vi "APU 1.4 In Place Output Read Structure.vi"(7 "Device outputs in":dbl[](array[numeric]), 8 "error in (no error)":errorcluster, 9 "FPGA ref in":T1, 11 "1.4 APU in":T4={"register names"={"shared settings"="", "input"="", "settings"="", "output"="", "go"="", "master"="", "send trigger"=""}, "shared settings"={"start"=0.0, "stuck limit"=0.0}, "settings"={"acceleration"=0.0, "enable accel"=FALSE}, "FIFO indexes"={"inputs"={"desired speed"=0, "reset"=0}, "outputs"={"crank angle"=0, "cycle angle"=0, "actual speed"=0, "devices synchronized"=0, "deviation error"=0}}, "input"={"desired speed"=0.0, "reset"=TRUE}, "degrees of 1 cycle u16"=0.0, "degrees of 1 crank u16"=0.0, "max deviation angle"=0.0}) -> (0 "error out":errorcluster, 1 "FPGA ref out":T1, 3 "1.4 APU out":T4={"register names"={"shared settings"="", "input"="", "settings"="", "output"="", "go"="", "master"="", "send trigger"=""}, "shared settings"={"start"=0.0, "stuck limit"=0.0}, "settings"={"acceleration"=0.0, "enable accel"=FALSE}, "FIFO indexes"={"inputs"={"desired speed"=0, "reset"=0}, "outputs"={"crank angle"=0, "cycle angle"=0, "actual speed"=0, "devices synchronized"=0, "deviation error"=0}}, "input"={"desired speed"=0.0, "reset"=TRUE}, "degrees of 1 cycle u16"=0.0, "degrees of 1 crank u16"=0.0, "max deviation angle"=0.0}, 5 "Device outputs out":dbl[](array[numeric]))   [LabVIEW 2020, in "Engine Simulation Toolkit Engine.lvlib"]
uses:
  Engine Simulation Toolkit Engine.lvlib
  Shared/1.4 APU Engine Data.ctl
  Shared/1.4 APU Engine FIFO Idxs.ctl
  APU 1.0 Run Refs.ctl
  APU 1.0 Output Ref.ctl
  APU 1.0 Input Ref.ctl
  Shared/Engine Simulation Toolkit Shared.lvlib
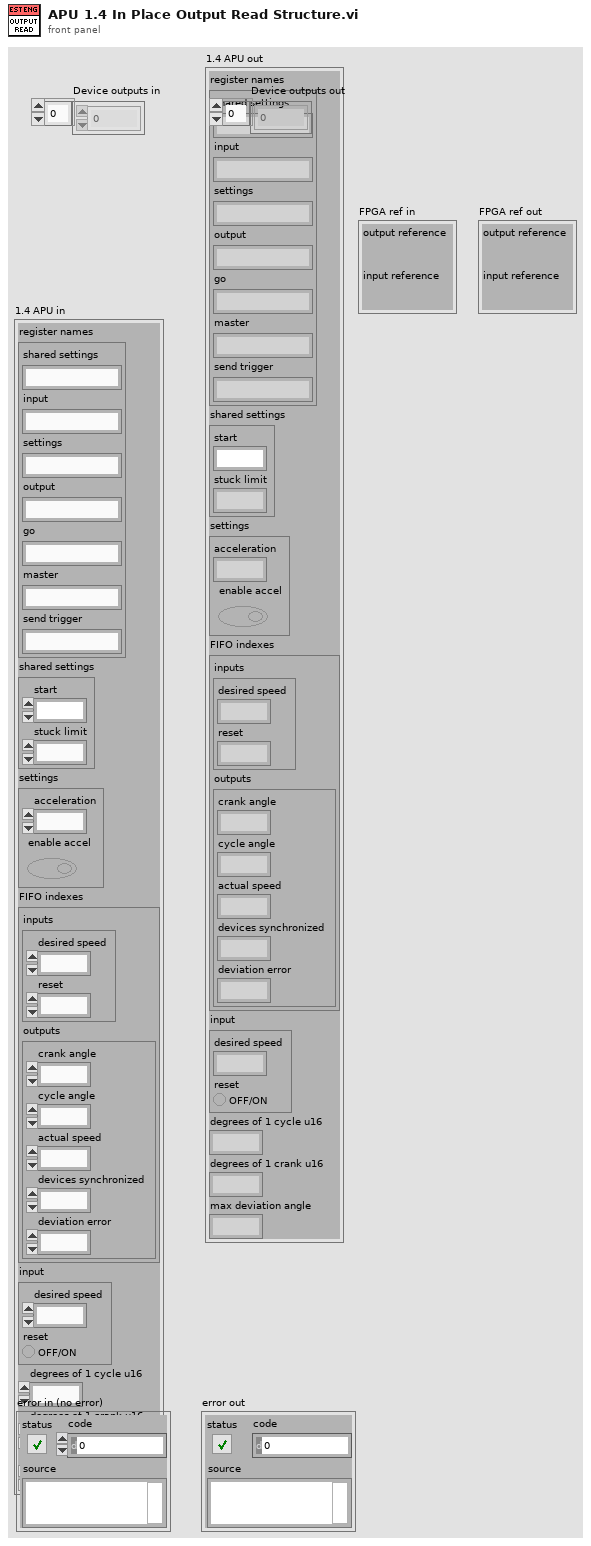
[diagram p1: front panel]
types:
  T1 = typedef "Engine Simulation Toolkit Engine.lvlib/APU 1.0 Run Refs.ctl" = cluster{"output reference":T2, "input reference":T3}
  T2 = typedef "Engine Simulation Toolkit Engine.lvlib/APU 1.0 Output Ref.ctl" = refnum<k20>
  T3 = typedef "Engine Simulation Toolkit Engine.lvlib/APU 1.0 Input Ref.ctl" = refnum<k20>
  T4 = typedef "Engine Simulation Toolkit Shared.lvlib/1.4 APU Engine Data.ctl" = cluster{"register names":cluster{"shared settings":string, "input":string, "settings":string, "output":string, "go":string, "master":string, "send trigger":string}, "shared settings":cluster{"start":fxp<+,17,17>, "stuck limit":fxp<+,18,18>}, "settings":cluster{"acceleration":fxp<+,18,-20>, "enable accel":bool}, "FIFO indexes":T5, "input":cluster{"desired speed":fxp<+/-,23,2>, "reset":bool}, "degrees of 1 cycle u16":dbl, "degrees of 1 crank u16":dbl, "max deviation angle":dbl}
  T5 = typedef "Engine Simulation Toolkit Shared.lvlib/1.4 APU Engine FIFO Idxs.ctl" = cluster{"inputs":cluster{"desired speed":i32, "reset":i32}, "outputs":cluster{"crank angle":i32, "cycle angle":i32, "actual speed":i32, "devices synchronized":i32, "deviation error":i32}}
  T6 = cluster{"crank angle":i32, "cycle angle":i32, "actual speed":i32, "devices synchronized":i32, "deviation error":i32}
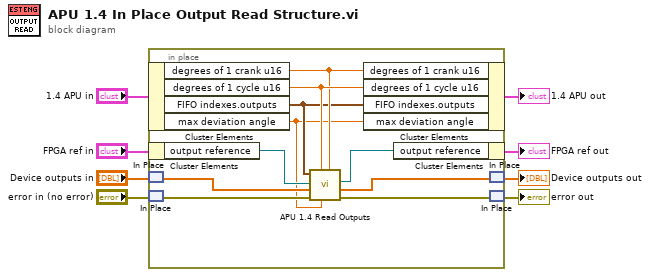
[diagram p0: block diagram]
diagram:
  n1 = in-place {
    n2 = in-place-cluster #1("1.4 APU in") -> ("degrees of 1 crank u16"=w13:dbl, "degrees of 1 cycle u16"=w14:dbl, "FIFO indexes.outputs"=w10:T6, "max deviation angle"=w9:dbl)
    n3 = in-place-cluster #2("FPGA ref in") -> ("output reference"=w12:T2)
    n4 = in-place-match #3("Device outputs in") -> (w16:dbl[])
    n5 = in-place-match #4("error in (no error)") -> (w18:errorcluster)
    n6 = call "APU 1.4 Read Outputs.vi"("degrees of 1 crank u16"=w13, "max deviation angle"=w9, "degrees of 1 cycle u16"=w14, "error in (no error)"=w18, "Device outputs in"=w16, "output reference in"=w12, "FIFO indexes.outputs"=w10) -> ("error out"=w17:errorcluster, "Device outputs out"=w15:dbl[], "output reference out"=w11:T2)  [unwired: 2 in]
    n7 = in-place-cluster #1("degrees of 1 crank u16"=w13, "degrees of 1 cycle u16"=w14, "FIFO indexes.outputs"=w10, "max deviation angle"=w9) -> (→"1.4 APU out":T4)
    n8 = in-place-cluster #2("output reference"=w11) -> (→"FPGA ref out":T1)
    n9 = in-place-match #3(w15) -> (→"Device outputs out":dbl[])
    n10 = in-place-match #4(w17) -> (→"error out":errorcluster)
  }
